vi "AdamsEncoder.vi"(6 "DiffConstant":dbl=300.0, 8 "Change each time":dbl=1e-09, 10 "FW2Rate":dbl, 11 "FW1Rate":dbl) -> (2 "FW2Change":dbl, 3 "FW1Change":dbl)   [LabVIEW 2014]
panel:
  in  "OffSetState":T1(ring)
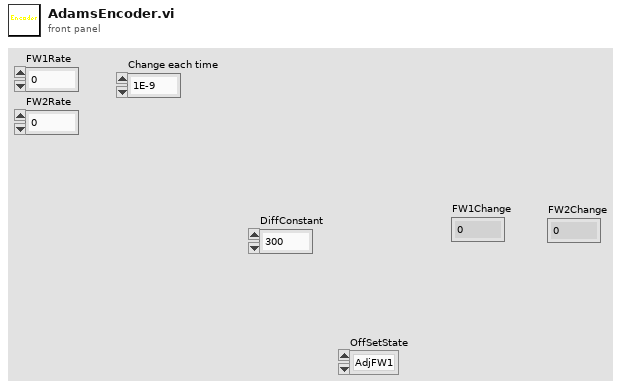
[diagram p1: front panel]
types:
  T1 = enum16{"AdjFW1", "AdjFW2", "FW2H", "FW1H", "Equal"}
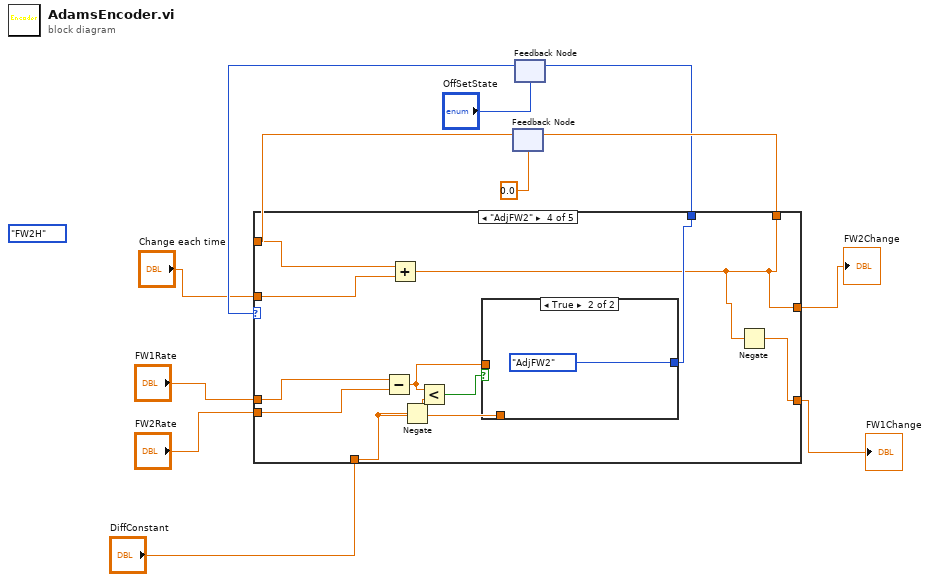
[diagram p0: block diagram]
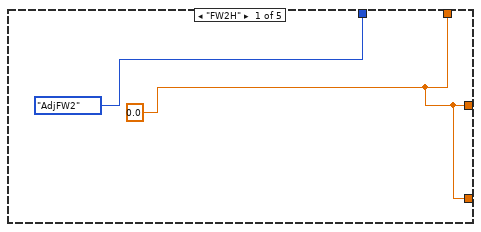
[diagram p2: hidden frame]
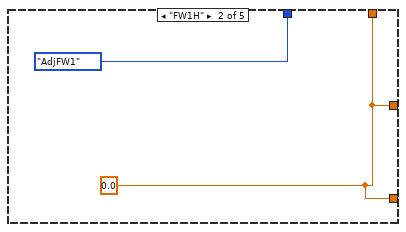
[diagram p3: hidden frame]
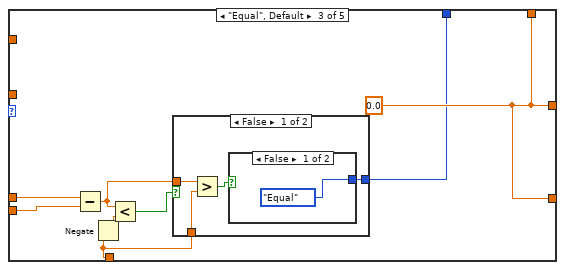
[diagram p4: hidden frame]
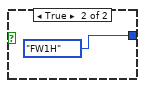
[diagram p5: hidden frame]
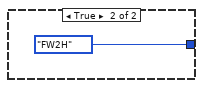
[diagram p6: hidden frame]
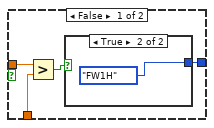
[diagram p7: hidden frame]
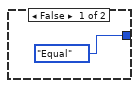
[diagram p8: hidden frame]
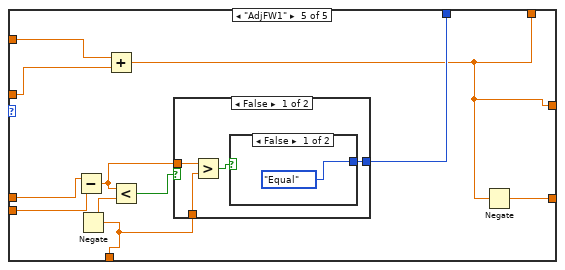
[diagram p9: hidden frame]
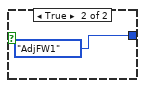
[diagram p10: hidden frame]
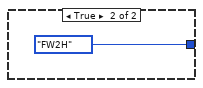
[diagram p11: hidden frame]
diagram:
  (unwired) T1."FW2H" ("OffSetState")
  n1 = feedback #1(0.0) -> (w9:dbl)
  n2 = feedback #2("OffSetState") -> (w6:T1)
  n3 = case shown="\"AdjFW2\"" w6 {
    tunnel: [w14 w16 w24 w33 w52] -> w12
    tunnel: [w14 w16 w24 w35 w51] -> w11
    tunnel: w9 -> [_ _ _ w34 w53]
    tunnel: [w14 w16 w24 w33 w52] -> w8
    tunnel: "FW1Rate" -> [_ _ w23 w39 w57]
    tunnel: "FW2Rate" -> [_ _ w22 w38 w56]
    tunnel: "DiffConstant" -> [_ _ w18 w37 w55]
    tunnel: [T1."AdjFW2" ("OffSetState") T1."AdjFW1" ("OffSetState") w17 w36 w54] -> w4
    tunnel: "Change each time" -> [_ _ _ w32 w50]
    frame "FW2H" {
      w14 = 0.0
    }
    frame "FW1H" {
      w16 = 0.0
    }
    frame "Equal", Default {
      w24 = 0.0
      n4 = Subtract(x=w23, y=w22) -> (x-y=w20:dbl)
      n5 = Negate(x=w18) -> (-x=w19:dbl)
      n6 = Less?(x=w20, y=w19) -> (x < y?=w21:bool)
      n7 = case shown="False" w21 {
        tunnel: w20 -> [w27 _]
        tunnel: w18 -> [w26 _]
        tunnel: [w25 T1."FW2H" ("OffSetState")] -> w17
        frame False {
          n8 = Greater?(x=w27, y=w26) -> (0:w28:bool)
          n9 = case shown="False" w28 {
            tunnel: [T1."Equal" ("OffSetState") T1."FW1H" ("OffSetState")] -> w25
            frame False {
            }
            frame True {
            }
          }
        }
        frame True {
        }
      }
    }
    frame "AdjFW2" {
      n10 = Subtract(x=w39, y=w38) -> (x-y=w41:dbl)
      n11 = Add(x=w34, y=w32) -> (x+y=w33:dbl)
      n12 = Negate(x=w37) -> (-x=w40:dbl)
      n13 = Less?(x=w41, y=w40) -> (x < y?=w42:bool)
      n14 = case shown="True" w42 {
        tunnel: w41 -> [w45 _]
        tunnel: w37 -> [w44 _]
        tunnel: [w43 T1."AdjFW2" ("OffSetState")] -> w36
        frame False {
          n15 = Greater?(x=w45, y=w44) -> (0:w46:bool)
          n16 = case shown="True" w46 {
            tunnel: [T1."Equal" ("OffSetState") T1."FW1H" ("OffSetState")] -> w43
            frame False {
            }
            frame True {
            }
          }
        }
        frame True {
        }
      }
      n17 = Negate(x=w33) -> (-x=w35:dbl)
    }
    frame "AdjFW1" {
      n18 = Subtract(x=w57, y=w56) -> (x-y=w59:dbl)
      n19 = Negate(x=w55) -> (-x=w58:dbl)
      n20 = Add(x=w53, y=w50) -> (x+y=w52:dbl)
      n21 = Less?(x=w59, y=w58) -> (x < y?=w60:bool)
      n22 = case shown="False" w60 {
        tunnel: w59 -> [w63 _]
        tunnel: w55 -> [w62 _]
        tunnel: [w61 T1."FW2H" ("OffSetState")] -> w54
        frame False {
          n23 = Greater?(x=w63, y=w62) -> (0:w64:bool)
          n24 = case shown="False" w64 {
            tunnel: [T1."Equal" ("OffSetState") T1."AdjFW1" ("OffSetState")] -> w61
            frame False {
            }
            frame True {
            }
          }
        }
        frame True {
        }
      }
      n25 = Negate(x=w52) -> (-x=w51:dbl)
    }
  }
  "FW1Change" <- w11
  "FW2Change" <- w12
  n26 = feedback-in #1(w8) -> ()
  n27 = feedback-in #2(w4) -> ()
